vi "getStatus.vi"() -> (0 "framesInMemory":u16, 1 "statusFlags":u8, 2 "return type":i32)   [LabVIEW 2012]
uses:
  hidapi_32bits.dll
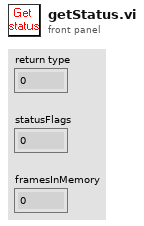
[diagram p1: front panel]
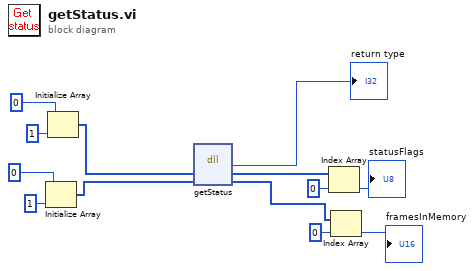
[diagram p0: block diagram]
diagram:
  n1 = Initialize Array(u16 0 ("element"), 1 ("dimension size")) -> (w8:u16[])
  n2 = Initialize Array(u8 0 ("element"), 1 ("dimension size")) -> (w9:u8[])
  n3 = dll-call lib="C:/All_Data/mikrocont/Project1/New_controller__Jan_2015/LabView_Aug_2015/hidapi_32bits.dll" fn="getStatus"("statusFlags"=w9, "framesInMemory"=w8) -> ("return type"=→"return type":i32, "statusFlags"=w4:u8[], "framesInMemory"=w3:u16[])  [unwired: 3 in, 2 out]
  n4 = Index Array(array=w4, index=0) -> (element=→"statusFlags":u8)
  n5 = Index Array(array=w3, index=0) -> (element=→"framesInMemory":u16)
